vi "Read Air Low Temperature Limit.vi"(8 "error in (no error)":errorcluster, 11 "VISA resource name":refnum<visa-resource-name>) -> (0 "error out":errorcluster, 1 "Air Low Temperature Limit, C":dbl, 3 "VISA resource name out":refnum<visa-resource-name>)   [LabVIEW 2012, in "Temptronic TP04300.lvlib"]
doc: "This VI reads <b>Air Low Temperature Limit</b> in Celsius.\n\nDefault Value: -99.0\nValid Range: -99.9 - 25.0"
uses:
  <instrlib>/Temptronic TP04300/Temptronic TP04300.lvlib
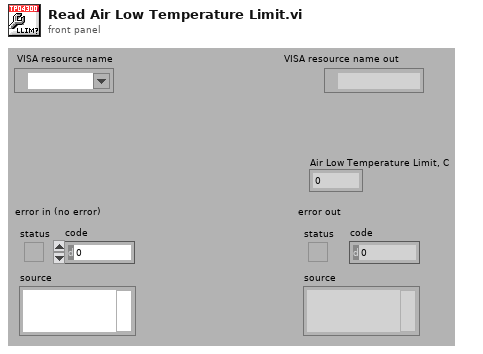
[diagram p1: front panel]
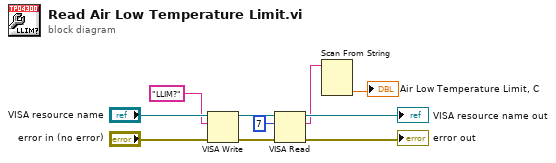
[diagram p0: block diagram]
diagram:
  n1 = VISA Write(VISA resource name="VISA resource name", write buffer="LLIM?" ("format string"), error in (no error)="error in (no error)") -> (VISA resource name out=w8:refnum<visa-resource-name>, error out=w7:errorcluster)  [unwired: 1 out]
  n2 = VISA Read(VISA resource name=w8, byte count=u32 7, error in (no error)=w7) -> (VISA resource name out=→"VISA resource name out":refnum<visa-resource-name>, read buffer=w3:string, error out=→"error out":errorcluster)  [unwired: 1 out]
  n3 = Scan From String(input string=w3) -> (output 1=→"Air Low Temperature Limit, C":dbl)  [unwired: 4 in, 3 out]
